vi "EditorPDF setRefnum.vi"(8 "error in (no error)":errorcluster, 10 "Refnum":T1, 11 "CreatePDF in":refnum<class "CreatePDF.lvclass">) -> (0 "error out":errorcluster, 3 "CreatePDF out":refnum<class "CreatePDF.lvclass">)   [LabVIEW 2018, in "CreatePDF.lvclass"]
uses:
  CreatePDF.lvclass
  CreatePDF.lvclass/CreatePDF.ctl
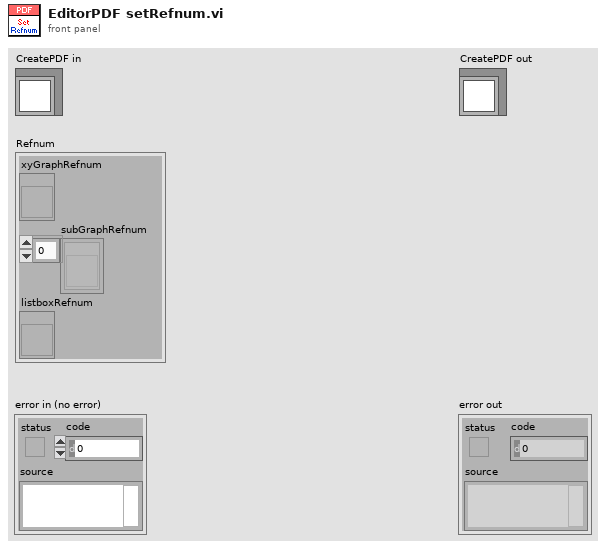
[diagram p1: front panel]
types:
  T1 = cluster{"xyGraphRefnum":refnum<vi>, "subGraphRefnum":refnum<vi>[], "listboxRefnum":refnum<vi>}
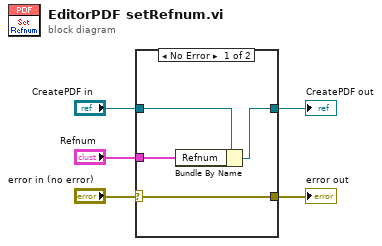
[diagram p0: block diagram]
diagram:
  n1 = case shown="No Error" "error in (no error)" {
    selector: "error in (no error)" -> [w9 w11]
    tunnel: [w9 w11] -> w4
    tunnel: [w6 w10] -> w2
    tunnel: "CreatePDF in" -> [w8 w10]
    tunnel: "Refnum" -> [w7 _]
    frame No Error {
      n2 = Bundle By Name(cluster=w8, "Refnum"=w7) -> (w6:refnum<class "CreatePDF.lvclass">)
    }
    frame Error {
    }
  }
  "error out" <- w4
  "CreatePDF out" <- w2
